vi "acknowledgeIRQ.vi"(8 "error in (no error)":errorcluster, 10 "IRQs":i32[](array[numeric]), 11 "OuterLoopClockIRQ in":refnum<class "OuterLoopClockIRQ.lvclass">) -> (0 "error out":errorcluster, 3 "OuterLoopClockIRQ out":refnum<class "OuterLoopClockIRQ.lvclass">)   [LabVIEW 2016, in "OuterLoopClockIRQ.lvclass"]
uses:
  OuterLoopClockIRQ.lvclass
  OuterLoopClockIRQ.lvclass/OuterLoopClockIRQ.ctl
  FPGA/FPGA.lvclass
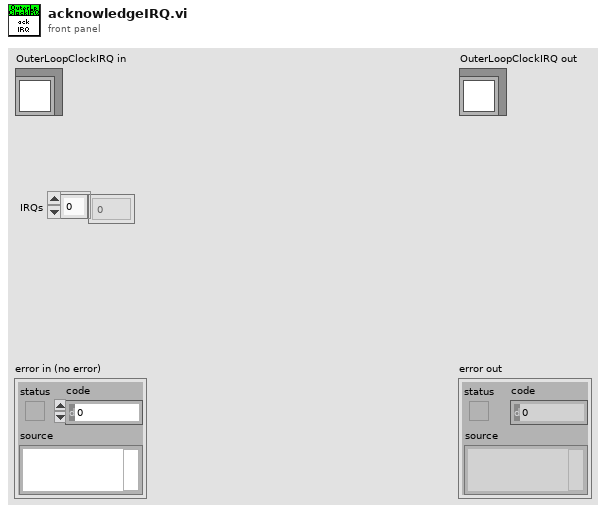
[diagram p1: front panel]
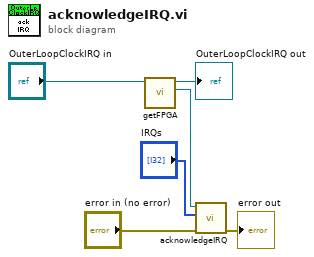
[diagram p0: block diagram]
diagram:
  n1 = call "getFPGA.vi"("OuterLoopClockIRQ in"="OuterLoopClockIRQ in") -> ("FPGA"=w6:refnum<class "FPGA.lvclass">, "OuterLoopClockIRQ out"=→"OuterLoopClockIRQ out":refnum<class "OuterLoopClockIRQ.lvclass">)  [unwired: 9 in]
  n2 = call "acknowledgeIRQ.vi"("error in (no error)"="error in (no error)", "IRQs"="IRQs", "FPGA in"=w6) -> ("error out"=→"error out":errorcluster)  [unwired: 7 in, 1 out]
